vi "事件结构的使用(下).vi"() -> ()   [LabVIEW 2018]
panel:
  in  "不是":bool
  in  "是":bool
  out "字符串":string="自学网是学习的好帮手吗？"
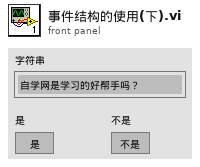
[diagram p1: front panel]
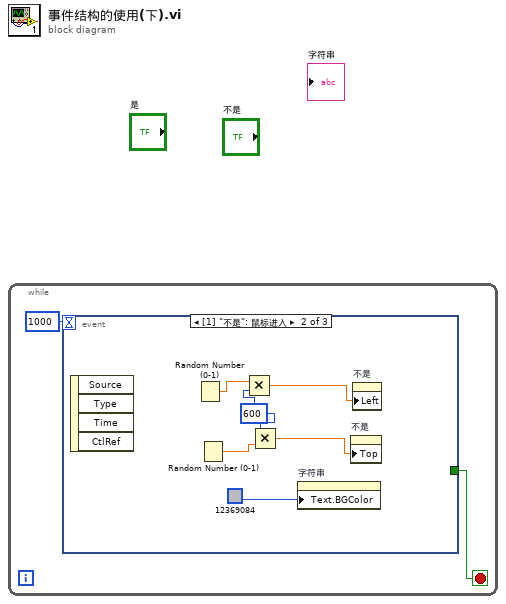
[diagram p0: block diagram]
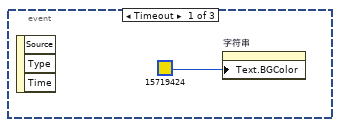
[diagram p2: hidden frame]
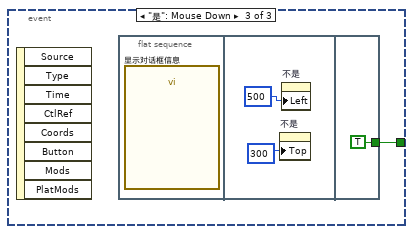
[diagram p3: hidden frame]
diagram:
  n1 = while {
    stop <- w2 stop-if-true
    n2 = event shown="[1] \"不是\": 鼠标进入" {
      selector: _ -> [_ _ _]
      dyn-events: _ -> [_ _ _]
      timeout: 1000 -> [_ _ _]
      tunnel: [_ _ w10] -> w2
      event Timeout {
        n3 = event-data() -> ()  [unwired: 1 in, 3 out]
        n4 = property on="字符串" class="Str"("Text.BGColor"=u32 15719424) -> ()  [unwired: 2 in, 2 out]
      }
      event "不是": Mouse Enter {
        w9 = 600
        n5 = event-data() -> ()  [unwired: 1 in, 4 out]
        n6 = Random Number (0-1)() -> (number: 0 to 1=w7:dbl)
        n7 = Random Number (0-1)() -> (number: 0 to 1=w8:dbl)
        n8 = Multiply(x=w7, y=w9) -> (x*y=w6:dbl)
        n9 = Multiply(x=w9, y=w8) -> (x*y=w5:dbl)
        n10 = property on="字符串" class="Str"("Text.BGColor"=u32 12369084) -> ()  [unwired: 2 in, 2 out]
        n11 = property on="不是" class="Bool"("Top"=w5) -> ()  [unwired: 2 in, 2 out]
        n12 = property on="不是" class="Bool"("Left"=w6) -> ()  [unwired: 2 in, 2 out]
      }
      event "是": Mouse Down {
        n13 = event-data() -> ()  [unwired: 1 in, 8 out]
        n14 = flat-sequence {
          tunnel: [TRUE] -> w10
          frame #0 {
            n15 = call "显示对话框信息"() -> ()  [unwired: 10 in, 2 out]
          }
          frame #1 {
            n16 = property on="不是" class="Bool"("Top"=300) -> ()  [unwired: 2 in, 2 out]
            n17 = property on="不是" class="Bool"("Left"=500) -> ()  [unwired: 2 in, 2 out]
          }
          frame #2 {
          }
        }
      }
    }
  }
